vi "ZDataVIS_Update_Cursor_SingleArrayTest.vi"(7 "Field/Temperature 2":refnum<vi>, 8 "error in (no error)":errorcluster, 9 "Cursor Graph":refnum<vi>, 10 "update bool":refnum<vi>, 11 "State Wire IN 2":T1={"Core"={"Current VI Reference"=refnum, "Close Panel on Exit?"=FALSE}, "Channel DVRs"=[], "Sweep Data Cluster"={"Vfast"=[[0.0, 0.25, 0.5, 0.75, 1.0, 1.25, 1.5, 1.75, 2.0, 2.25, 2.5, 2.75, 3.0, 3.25, 3.5, 3.75, 4.0, 4.25, 4.5, 4.75, 5.0, 5.25, 5.5, 5.75, 6.0, 6.25, 6.5, 6.75, 7.0, 7.25, 7.5, 7.75, 8.0, 8.25, 8.5, 8.75, 9.0, 9.25, 9.5, 9.75, 10.0, 10.25, 10.5, 10.75, 11.0, 11.25, 11.5, 11.75, 12.0, 12.25, 12.5, 12.75, 13.0, 13.25, 13.5, 13.75, 14.0, 14.25, 14.5, 14.75, 15.0]], "Vslow"=[0.0, 1.0, 2.0, 3.0, 4.0, 5.0, 6.0, 7.0], "Vslowest"=[7.00003046875], "Comments"="      #Vslow/#Vfast/# of IV curves/BT offset/#discarded IV curves/Manual offset:\n /8/61/1/0/0/0    \n#of fields: 1    \nField period 1 \nDecimate point 1.000000 \nScan names \nDAQ_Vbg\nB\nB \n IGOR\nX// Date: 7/19/2018 6:19 PM\nX// SA03008H\nX// \nX// Source 2 Drain 28 (lockin 1 and 7)\nX// Gohm resistor, sweep BG\nX// \nX// 50mV AC -150mV DC for the IV sweep\nX// \nX// 0 to 15 slowly at 0.25 V step sizes\nX// Stepping B 0-7 @ 1T steps\n\nX// B_Field=7.000000\n\nX// \n\nX// B_Field_Rate=0.400000\n\nX// \n\nX// DAQ_Vbg=15.000000\n\nX// \nX// B= 7.000030\n\n\n\n\n\n\n\n\n\n\n\n\n\n\n\n\n\n\n\n\n\n\n\n\n\n\n\n\n\n\n\n\n\n\n\n\n\n\n\n\nX \nX Display/R 'time.SA03008H.20180718.000487'\nX AppendToGraph 'temp.SA03008H.20180718.000487'\nX AppendToGraph 'B.SA03008H.20180718.000487'\nX AppendToGraph 'Vsource.SA03008H.20180718.000487'\nX AppendToGraph 'Lockin0.SA03008H.20180718.000487'\nX AppendToGraph 'Lockin1.SA03008H.20180718.000487'\nX AppendToGraph 'Lockin2.SA03008H.20180718.000487'\nX AppendToGraph 'Lockin3.SA03008H.20180718.000487'\nX AppendToGraph 'Lockin4.SA03008H.20180718.000487'\nX AppendToGraph 'Lockin5.SA03008H.20180718.000487'\nX AppendToGraph 'B_rate.SA03008H.20180718.000487'\nX AppendToGraph 'DC0.SA03008H.20180718.000487'\nX AppendToGraph 'DC1.SA03008H.20180718.000487'\nX AppendToGraph 'DC2.SA03008H.20180718.000487'\nX AppendToGraph 'DC3.SA03008H.20180718.000487'\nX AppendToGraph 'DC4.SA03008H.20180718.000487'\nX AppendToGraph 'DC5.SA03008H.20180718.000487'\nX AppendToGraph 'DC6.SA03008H.20180718.000487'\nX AppendToGraph 'DC7.SA03008H.20180718.000487'\nX Label bottom \"x label\"\nX Label left \"y label\"\nX ModifyGraph rgb('time.SA03008H.20180718.000487')=(65280,0,0)\nX ModifyGraph rgb('temp.SA03008H.20180718.000487')=(65280,18432,0)\nX ModifyGraph rgb('B.SA03008H.20180718.000487')=(65280,36864,0)\nX ModifyGraph rgb('Vsource.SA03008H.20180718.000487')=(65280,55296,0)\nX ModifyGraph rgb('Lockin0.SA03008H.20180718.000487')=(57344,65280,0)\nX ModifyGraph rgb('Lockin1.SA03008H.20180718.000487')=(37376,65280,0)\nX ModifyGraph rgb('Lockin2.SA03008H.20180718.000487')=(18944,65280,0)\nX ModifyGraph rgb('Lockin3.SA03008H.20180718.000487')=(512,65280,0)\nX ModifyGraph rgb('Lockin4.SA03008H.20180718.000487')=(0,65280,17920)\nX ModifyGraph rgb('Lockin5.SA03008H.20180718.000487')=(0,65280,36352)\nX ModifyGraph rgb('B_rate.SA03008H.20180718.000487')=(0,65280,54784)\nX ModifyGraph rgb('DC0.SA03008H.20180718.000487')=(0,57856,65280)\nX ModifyGraph rgb('DC1.SA03008H.20180718.000487')=(0,39424,65280)\nX ModifyGraph rgb('DC2.SA03008H.20180718.000487')=(0,20992,65280)\nX ModifyGraph rgb('DC3.SA03008H.20180718.000487')=(0,2560,65280)\nX ModifyGraph rgb('DC4.SA03008H.20180718.000487')=(17408,0,65280)\nX ModifyGraph rgb('DC5.SA03008H.20180718.000487')=(35840,0,65280)\nX ModifyGraph rgb('DC6.SA03008H.20180718.000487')=(54272,0,65280)\nX ModifyGraph rgb('DC7.SA03008H.20180718.000487')=(65280,0,58368)\nX Legend/C/N=text0/J \"\\\\s('time.SA03008H.20180718.000487') time\\r\\\\s('temp.SA03008H.20180718.000487') temp\\r\\\\s('B.SA03008H.20180718.000487') B\\r\\\\s('Vsource.SA03008H.20180718.000487') Vsource\\r\\\\s('Lockin0.SA03008H.20180718.000487') Lockin0\\r\\\\s('Lockin1.SA03008H.20180718.000487') Lockin1\\r\\\\s('Lockin2.SA03008H.20180718.000487') Lockin2\\r\\\\s('Lockin3.SA03008H.20180718.000487') Lockin3\\r\\\\s('Lockin4.SA03008H.20180718.000487') Lockin4\\r\\\\s('Lockin5.SA03008H.20180718.000487') Lockin5\\r\\\\s('B_rate.SA03008H.20180718.000487') B_rate\\r\\\\s('DC0.SA03008H.20180718.000487') DC0\\r\\\\s('DC1.SA03008H.20180718.000487') DC1\\r\\\\s('DC2.SA03008H.20180718.000487') DC2\\r\\\\s('DC3.SA03008H.20180718.000487') DC3\\r\\\\s('DC4.SA03008H.20180718.000487') DC4\\r\\\\s('DC5.SA03008H.20180718.000487') DC5\\r\\\\s('DC6.SA03008H.20180718.000487') DC6\\r\\\\s('DC7.SA03008H.20180718.000487') DC7\"\nX ModifyGraph mirror(bottom)=1\nX ModifyGraph width=216\nX ModifyGraph height={Aspect,0.6}\nX ModifyGraph Log(bottom)=0\nX ModifyGraph Log(left)=0\nX \n", "Scan names"=["DAQ_Vbg", "B", "B"]}, "Cursor Info"={"Fast Index"=[33.0, 33.0, 33.0, 33.0, 33.0, 33.0, 33.0, 33.0], "Slow Index"=4.0, "Slow Indices"=[0.0, 1.0, 2.0, 3.0, 4.0, 5.0, 6.0, 7.0], "Raw Cursor Position"={"X"=8.146964856230031, "Y"=4.108108108108109}, "Field / temp"=0}, "Scan names"=["DAQ_Vbg", "B", "B"], "Decimated X values"=[], "X Step Info"={"X Low"=-0.1, "X High"=0.1, "X Step"=4e-05}, "Voffset -2T"=0.0, "Wiring Configuration "=[], "Intensity Info DVR"=refnum, "Object RefNum"=refnum, "All Lockin AO DVR"=refnum, "itx # info"=[], "root processed directory"=path ""} {"X Step Info"."X Step" format="%#_6p"; "X Step Info"."X High" format="%#_6p"; "X Step Info"."X Low" format="%#_6p"}) -> (0 "error out":errorcluster, 1 "Field":dbl=4.108108108108109, 2 "slowest":dbl=7.00003046875, 3 "State Wire IN 3":T1={"Core"={"Current VI Reference"=refnum, "Close Panel on Exit?"=FALSE}, "Channel DVRs"=[], "Sweep Data Cluster"={"Vfast"=[[0.0, 0.25, 0.5, 0.75, 1.0, 1.25, 1.5, 1.75, 2.0, 2.25, 2.5, 2.75, 3.0, 3.25, 3.5, 3.75, 4.0, 4.25, 4.5, 4.75, 5.0, 5.25, 5.5, 5.75, 6.0, 6.25, 6.5, 6.75, 7.0, 7.25, 7.5, 7.75, 8.0, 8.25, 8.5, 8.75, 9.0, 9.25, 9.5, 9.75, 10.0, 10.25, 10.5, 10.75, 11.0, 11.25, 11.5, 11.75, 12.0, 12.25, 12.5, 12.75, 13.0, 13.25, 13.5, 13.75, 14.0, 14.25, 14.5, 14.75, 15.0]], "Vslow"=[0.0, 1.0, 2.0, 3.0, 4.0, 5.0, 6.0, 7.0], "Vslowest"=[7.00003046875], "Comments"="      #Vslow/#Vfast/# of IV curves/BT offset/#discarded IV curves/Manual offset:\n /8/61/1/0/0/0    \n#of fields: 1    \nField period 1 \nDecimate point 1.000000 \nScan names \nDAQ_Vbg\nB\nB \n IGOR\nX// Date: 7/19/2018 6:19 PM\nX// SA03008H\nX// \nX// Source 2 Drain 28 (lockin 1 and 7)\nX// Gohm resistor, sweep BG\nX// \nX// 50mV AC -150mV DC for the IV sweep\nX// \nX// 0 to 15 slowly at 0.25 V step sizes\nX// Stepping B 0-7 @ 1T steps\n\nX// B_Field=7.000000\n\nX// \n\nX// B_Field_Rate=0.400000\n\nX// \n\nX// DAQ_Vbg=15.000000\n\nX// \nX// B= 7.000030\n\n\n\n\n\n\n\n\n\n\n\n\n\n\n\n\n\n\n\n\n\n\n\n\n\n\n\n\n\n\n\n\n\n\n\n\n\n\n\n\nX \nX Display/R 'time.SA03008H.20180718.000487'\nX AppendToGraph 'temp.SA03008H.20180718.000487'\nX AppendToGraph 'B.SA03008H.20180718.000487'\nX AppendToGraph 'Vsource.SA03008H.20180718.000487'\nX AppendToGraph 'Lockin0.SA03008H.20180718.000487'\nX AppendToGraph 'Lockin1.SA03008H.20180718.000487'\nX AppendToGraph 'Lockin2.SA03008H.20180718.000487'\nX AppendToGraph 'Lockin3.SA03008H.20180718.000487'\nX AppendToGraph 'Lockin4.SA03008H.20180718.000487'\nX AppendToGraph 'Lockin5.SA03008H.20180718.000487'\nX AppendToGraph 'B_rate.SA03008H.20180718.000487'\nX AppendToGraph 'DC0.SA03008H.20180718.000487'\nX AppendToGraph 'DC1.SA03008H.20180718.000487'\nX AppendToGraph 'DC2.SA03008H.20180718.000487'\nX AppendToGraph 'DC3.SA03008H.20180718.000487'\nX AppendToGraph 'DC4.SA03008H.20180718.000487'\nX AppendToGraph 'DC5.SA03008H.20180718.000487'\nX AppendToGraph 'DC6.SA03008H.20180718.000487'\nX AppendToGraph 'DC7.SA03008H.20180718.000487'\nX Label bottom \"x label\"\nX Label left \"y label\"\nX ModifyGraph rgb('time.SA03008H.20180718.000487')=(65280,0,0)\nX ModifyGraph rgb('temp.SA03008H.20180718.000487')=(65280,18432,0)\nX ModifyGraph rgb('B.SA03008H.20180718.000487')=(65280,36864,0)\nX ModifyGraph rgb('Vsource.SA03008H.20180718.000487')=(65280,55296,0)\nX ModifyGraph rgb('Lockin0.SA03008H.20180718.000487')=(57344,65280,0)\nX ModifyGraph rgb('Lockin1.SA03008H.20180718.000487')=(37376,65280,0)\nX ModifyGraph rgb('Lockin2.SA03008H.20180718.000487')=(18944,65280,0)\nX ModifyGraph rgb('Lockin3.SA03008H.20180718.000487')=(512,65280,0)\nX ModifyGraph rgb('Lockin4.SA03008H.20180718.000487')=(0,65280,17920)\nX ModifyGraph rgb('Lockin5.SA03008H.20180718.000487')=(0,65280,36352)\nX ModifyGraph rgb('B_rate.SA03008H.20180718.000487')=(0,65280,54784)\nX ModifyGraph rgb('DC0.SA03008H.20180718.000487')=(0,57856,65280)\nX ModifyGraph rgb('DC1.SA03008H.20180718.000487')=(0,39424,65280)\nX ModifyGraph rgb('DC2.SA03008H.20180718.000487')=(0,20992,65280)\nX ModifyGraph rgb('DC3.SA03008H.20180718.000487')=(0,2560,65280)\nX ModifyGraph rgb('DC4.SA03008H.20180718.000487')=(17408,0,65280)\nX ModifyGraph rgb('DC5.SA03008H.20180718.000487')=(35840,0,65280)\nX ModifyGraph rgb('DC6.SA03008H.20180718.000487')=(54272,0,65280)\nX ModifyGraph rgb('DC7.SA03008H.20180718.000487')=(65280,0,58368)\nX Legend/C/N=text0/J \"\\\\s('time.SA03008H.20180718.000487') time\\r\\\\s('temp.SA03008H.20180718.000487') temp\\r\\\\s('B.SA03008H.20180718.000487') B\\r\\\\s('Vsource.SA03008H.20180718.000487') Vsource\\r\\\\s('Lockin0.SA03008H.20180718.000487') Lockin0\\r\\\\s('Lockin1.SA03008H.20180718.000487') Lockin1\\r\\\\s('Lockin2.SA03008H.20180718.000487') Lockin2\\r\\\\s('Lockin3.SA03008H.20180718.000487') Lockin3\\r\\\\s('Lockin4.SA03008H.20180718.000487') Lockin4\\r\\\\s('Lockin5.SA03008H.20180718.000487') Lockin5\\r\\\\s('B_rate.SA03008H.20180718.000487') B_rate\\r\\\\s('DC0.SA03008H.20180718.000487') DC0\\r\\\\s('DC1.SA03008H.20180718.000487') DC1\\r\\\\s('DC2.SA03008H.20180718.000487') DC2\\r\\\\s('DC3.SA03008H.20180718.000487') DC3\\r\\\\s('DC4.SA03008H.20180718.000487') DC4\\r\\\\s('DC5.SA03008H.20180718.000487') DC5\\r\\\\s('DC6.SA03008H.20180718.000487') DC6\\r\\\\s('DC7.SA03008H.20180718.000487') DC7\"\nX ModifyGraph mirror(bottom)=1\nX ModifyGraph width=216\nX ModifyGraph height={Aspect,0.6}\nX ModifyGraph Log(bottom)=0\nX ModifyGraph Log(left)=0\nX \n", "Scan names"=["DAQ_Vbg", "B", "B"]}, "Cursor Info"={"Fast Index"=[33.0, 33.0, 33.0, 33.0, 33.0, 33.0, 33.0, 33.0], "Slow Index"=4.0, "Slow Indices"=[0.0, 1.0, 2.0, 3.0, 4.0, 5.0, 6.0, 7.0], "Raw Cursor Position"={"X"=8.146964856230031, "Y"=4.108108108108109}, "Field / temp"=0}, "Scan names"=["DAQ_Vbg", "B", "B"], "Decimated X values"=[], "X Step Info"={"X Low"=-0.1, "X High"=0.1, "X Step"=4e-05}, "Voffset -2T"=0.0, "Wiring Configuration "=[], "Intensity Info DVR"=refnum, "Object RefNum"=refnum, "All Lockin AO DVR"=refnum, "itx # info"=[], "root processed directory"=path ""} {"X Step Info"."X Step" format="%#_6p"; "X Step Info"."X High" format="%#_6p"; "X Step Info"."X Low" format="%#_6p"})   [LabVIEW 2016]
uses:
  ZDataVIS_StateWire.ctl
  <vilib>/Utility/miscctls.llb/LVPointDoubleTypeDef.ctl
  <userlib>/_OpenG.lib/dictionary/dictionary.llb/Dictionary Object RefNum__ogtk.ctl
  <userlib>/_OpenG.lib/dictionary/dictionary.llb/Dictionary Object RefNum - Enum__ogtk.ctl
panel:
  # "cursor x"
  # "cursor y"
  # "cursor x"
  # "cursor y"
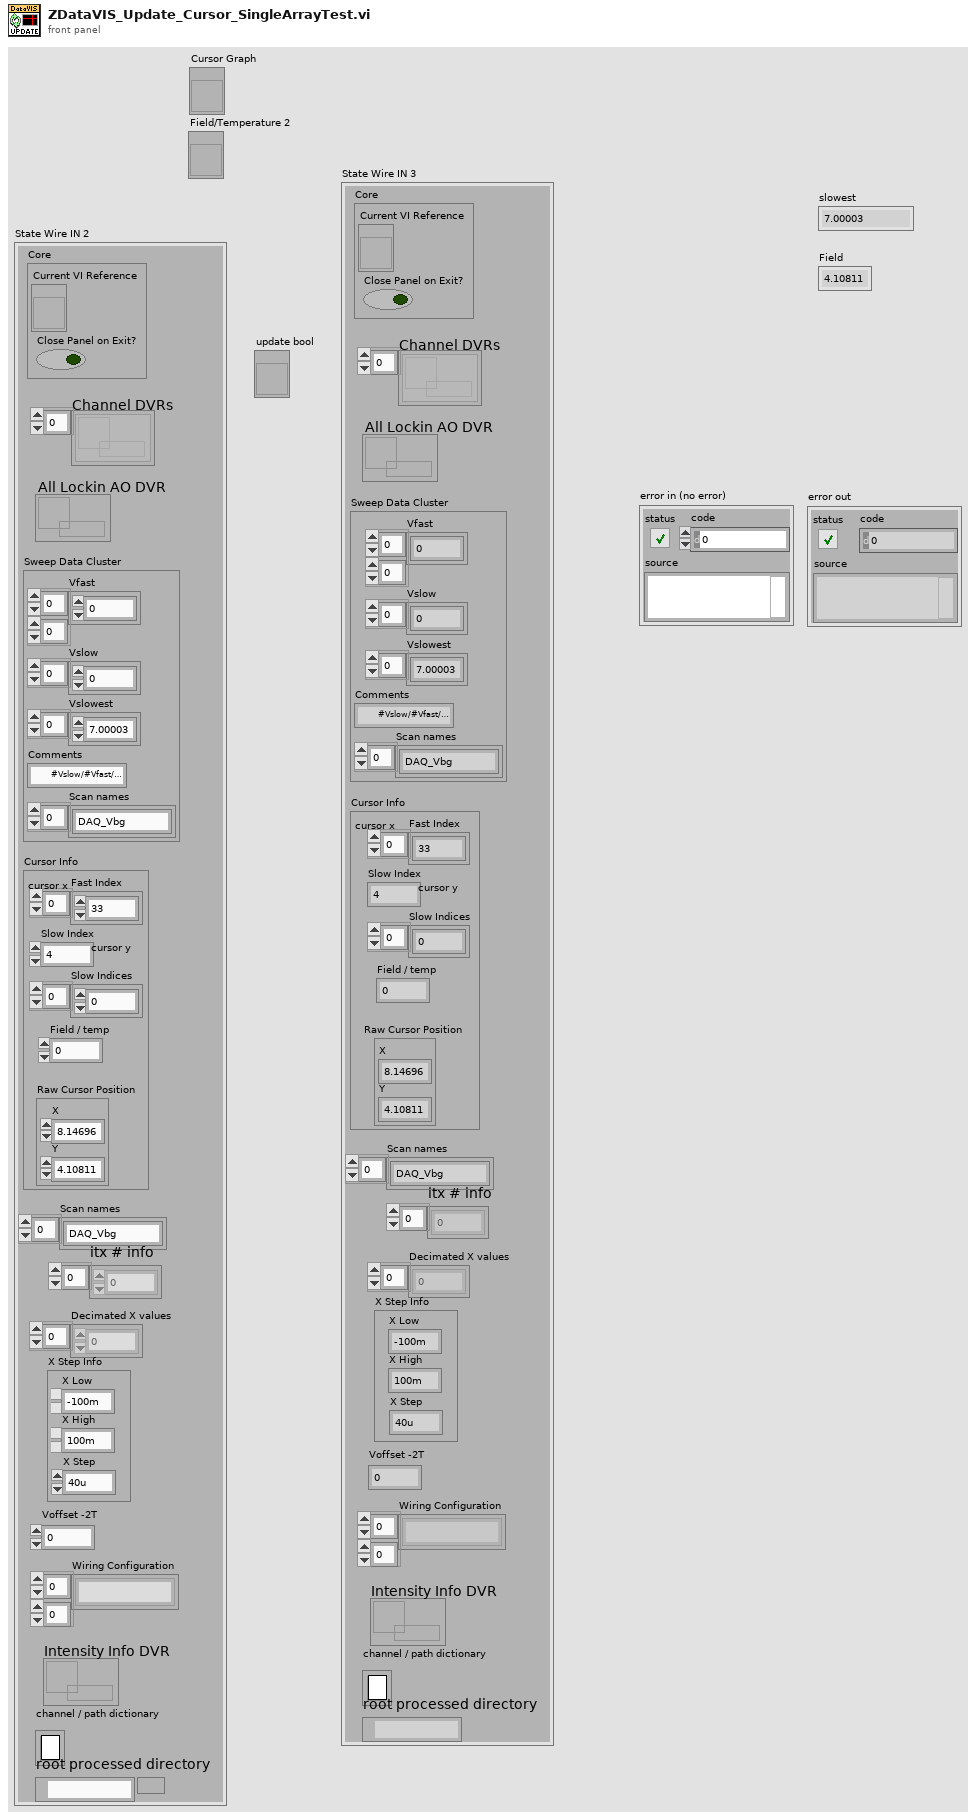
[diagram p1: front panel]
types:
  T1 = typedef "ZDataVIS_StateWire.ctl" = cluster{"Core":cluster{"Current VI Reference":refnum<vi>, "Close Panel on Exit?":bool}, "Channel DVRs":refnum<data-value>[], "Sweep Data Cluster":cluster{"Vfast":dbl[][], "Vslow":dbl[], "Vslowest":dbl[], "Comments":string, "Scan names":string[]}, "Cursor Info":cluster{"Fast Index":dbl[], "Slow Index":dbl, "Slow Indices":dbl[], "Raw Cursor Position":T2, "Field / temp":i32}, "Scan names":string[], "Decimated X values":dbl[], "X Step Info":cluster{"X Low":dbl, "X High":dbl, "X Step":dbl}, "Voffset -2T":dbl, "Wiring Configuration ":string[][], "Intensity Info DVR":refnum<data-value>, "Object RefNum":T3, "All Lockin AO DVR":refnum<data-value>, "itx # info":i32[], "root processed directory":path}
  T2 = typedef "LVPointDoubleTypeDef.ctl" = cluster{"X":dbl, "Y":dbl}
  T3 = typedef "Dictionary Object RefNum__ogtk.ctl" = refnum<k1>
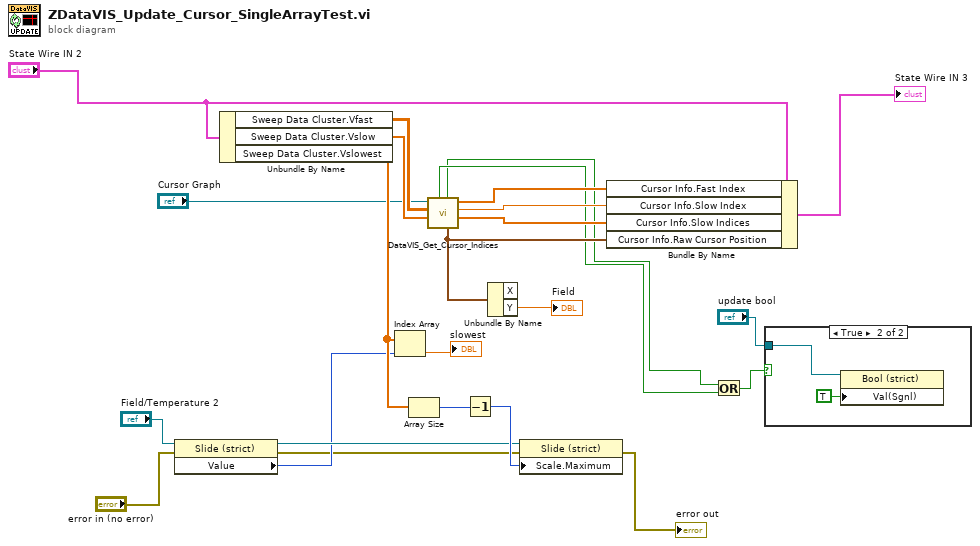
[diagram p0: block diagram]
diagram:
  n1 = property class="Slide (strict)"(reference="Field/Temperature 2", error in="error in (no error)") -> (error out=w6:errorcluster, "Value"=w8:i32)  [unwired: 1 out]
  n2 = Unbundle By Name("State Wire IN 2") -> ("Sweep Data Cluster.Vfast"=w23:dbl[][], "Sweep Data Cluster.Vslow"=w22:dbl[], "Sweep Data Cluster.Vslowest"=w17:dbl[])
  n3 = Index Array(array=w17, index=w8) -> (element=→"slowest":dbl)
  n4 = Array Size(array=w17) -> (size(s)=w21:i32)
  n5 = call "DataVIS_Get_Cursor_Indices.vi"("Vslow"=w22, "Vfast"=w23, "Cursor Graph"="Cursor Graph") -> ("Slow Indices"=w14:dbl[], "Slow Index (Cursor Y)"=w15:dbl, "Fast Index (Cursor X) (IDK why it's an array)"=w16:dbl[], "Raw Cursor Position"=w13:T2, "Fresh Y"=w2:bool, "Fresh X"=w3:bool)  [unwired: 2 in, 1 out]
  n6 = Decrement(x=w21) -> (x-1=w20:i32)
  n7 = Unbundle By Name(w13) -> ("Y"=→"Field":dbl)  [unwired: 1 out]
  n8 = property on="Property Node" class="Slide (strict)"(reference="Field/Temperature 2", error in=w6, "Scale.Maximum"=w20) -> (error out=→"error out":errorcluster)  [unwired: 1 out]
  n9 = Bundle By Name(cluster="State Wire IN 2", "Cursor Info.Fast Index"=w16, "Cursor Info.Slow Index"=w15, "Cursor Info.Slow Indices"=w14, "Cursor Info.Raw Cursor Position"=w13) -> (→"State Wire IN 3":T1)
  n10 = Or(x=w2, y=w3) -> (x .or. y?=w1:bool)
  n11 = case shown="True" w1 {
    tunnel: "update bool" -> [_ w24]
    frame False {
    }
    frame True {
      n12 = property class="Bool (strict)"(reference=w24, "Val(Sgnl)"=TRUE ("Value (Signaling)")) -> ()  [unwired: 1 in, 2 out]
    }
  }
